vi "Constants.vi"() -> ()   [LabVIEW 2027, in "Embedded Data Logger Shared.lvlib"]
doc: "Use this Global VI to access the GUIDs assigned to the page resources of the Custom Device."
uses:
  Embedded Data Logger Shared.lvlib
panel:
  in  "Tab Control":enum32{"GUIDs", "Constants", "Properties"}(tab)=enum."Properties"
  in  "Decimation GUID":string="e3467543-06b1-40b2-b868-415e5fc97bc1"
  in  "Embedded Data Logger Disabled GUID":string="d5523103-54a2-4b40-b917-a7ebcdb2735a"
  in  "Commands Group GUID":string="4f1afc32-5d3f-480b-ab1d-e879716c7d05"
  in  "Status Group GUID":string="a53a1349-a480-4f9e-9001-22192f2aa75f"
  in  "Channel Groups GUID":string="708d9ba3-288f-456f-bd58-8911c913706f"
  in  "Channel Group GUID":string="6f0afb90-3eee-463c-9817-5273ea7ccf5e"
  in  "File GUID":string="29edb790-3e4e-4121-9b93-a3d0540ab92c"
  in  "File Status GUID":string="0565a14b-6056-4bf2-ab89-d54684e64d40"
  in  "Command GUID":string="9b525fa0-4d4a-4ec1-902b-bfeef88ebbcc"
  in  "Trigger GUID":string="19ab609c-2807-4208-9214-1b9da8fe089c"
  in  "Embedded Data Logger GUID":string="382db339-b6fb-45a6-86c0-031bb1110bb1"
  in  "Additional Property Values":string="Additional Property Values"
  in  "Additional Property Names":string="Additional Property Names"
  in  "Append Waveform Properties":string="Append Waveform Properties"
  in  "Pretrigger Samples":string="Pretrigger Samples"
  in  "Pretrigger":string="Pretrigger"
  in  "Auto Open":string="Auto Open"
  in  "Segment Size":string="Segment Size"
  in  "Segment Files By":string="Segment Files By"
  in  "Segment Files":string="Segment Files"
  in  "Log Archive Dir":string="Log Archive Dir"
  in  "Archive Files":string="Archive Files"
  in  "Timestamp":string="Timestamp"
  in  "Log File Dir":string="Log File Dir"
  in  "Compiled.Settings":string="Compiled.Settings"
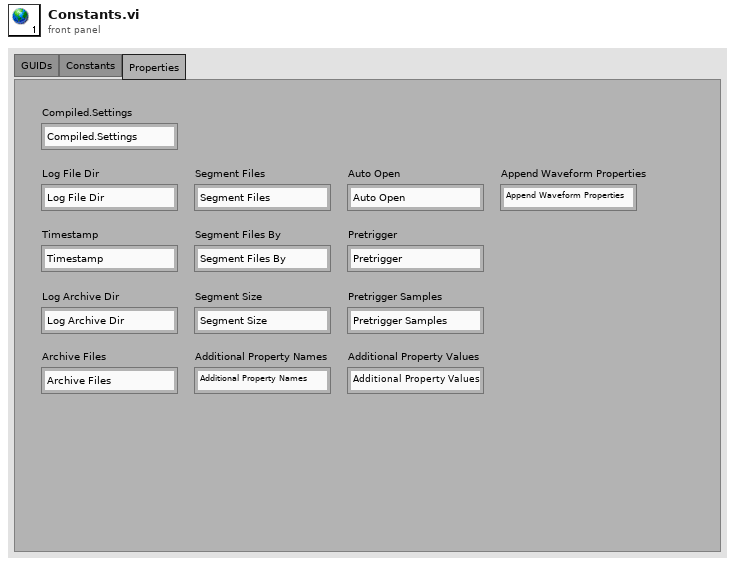
[diagram p1: front panel]
diagram:
